vi "Init Hardware.vi"(8 "error in (no error)":errorcluster, 11 "LabJack Driver in":refnum<class "LabJack Driver.lvclass">) -> (0 "error out":errorcluster, 3 "LabJack Driver out":refnum<class "LabJack Driver.lvclass">)   [LabVIEW 2021, in "LabJack Driver.lvclass"]
uses:
  LabJack Driver.lvclass
  C:/Git/NHMFL_Core/Libraries/Instruments/Instrument Driver/Instrument Driver.lvclass
  Instrument Driver/Instrument Driver.lvclass/Instrument Driver.ctl
  Instrument Driver/Read Recorder name.vi
  Instrument Driver/Write Channel names.vi
  Instrument Driver/Write Channel units.vi
  Simple VISA Reader/Simple VISA Reader Driver.lvclass
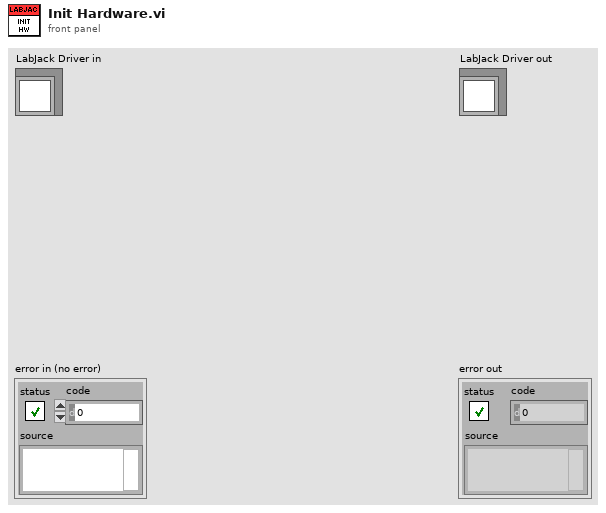
[diagram p1: front panel]
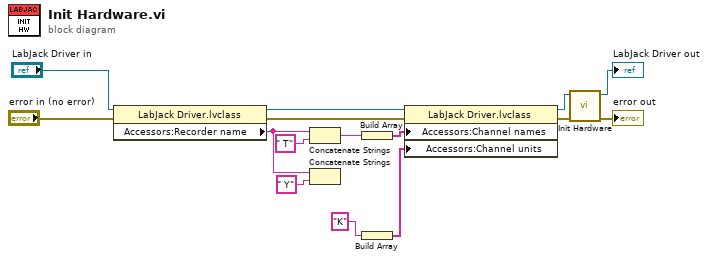
[diagram p0: block diagram]
diagram:
  n1 = property class="LabJack Driver.lvclass"(reference="LabJack Driver in", error in="error in (no error)") -> (reference out=w12:refnum<class "LabJack Driver.lvclass">, error out=w13:errorcluster, "Accessors:Recorder name"=w7:string)
  n2 = Concatenate Strings(w7, " T") -> (w8:string)
  n3 = Concatenate Strings(w7, " Y") -> ()  [unwired: 1 out]
  n4 = Build Array(w8) -> (w10:string[])
  n5 = Build Array("K") -> (w11:string[])
  n6 = property class="LabJack Driver.lvclass"(reference=w12, error in=w13, "Accessors:Channel names"=w10, "Accessors:Channel units"=w11) -> (reference out=w4:refnum<class "LabJack Driver.lvclass">, error out=w5:errorcluster)
  n7 = call-parent "Init Hardware.vi"("error in (no error)"=w5, "Instrument Driver in"=w4) -> ("error out"=→"error out":errorcluster, "Instrument Driver out"=→"LabJack Driver out":refnum<class "LabJack Driver.lvclass">)  [unwired: 8 in]
